vi "Initialize Queues.vi"(8 "error in":errorcluster) -> (0 "error out":errorcluster)   [LabVIEW 2019]
doc: "Initialize all queues.\n\n-----\nJuan Navarro\nLab it Studio"
uses:
  MHL/MHL.lvlib
  Modules/Deep Thought/Deep Thought.lvlib
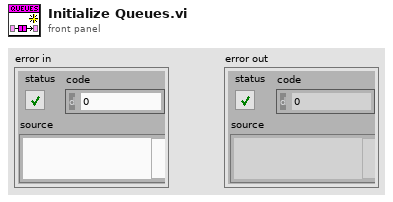
[diagram p1: front panel]
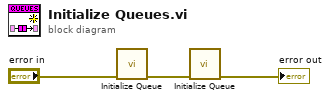
[diagram p0: block diagram]
diagram:
  n1 = call "Initialize Queue.vi"("error in"="error in") -> ("error out"=w2:errorcluster)  [unwired: 9 in, 1 out]
  n2 = call "Initialize Queue.vi"("error in"=w2) -> ("error out"=→"error out":errorcluster)  [unwired: 9 in, 1 out]
